vi "XY Graph Show-Hide Grid Event.vi"(8 "Error In":errorcluster, 11 "XYGraph in":T1) -> (0 "Error Out":errorcluster, 1 "Message":string)   [LabVIEW 2019, in "XY Graph Add-Ons.lvlib"]
uses:
  XY Graph Add-Ons.lvlib
  XY Graph Refnum.ctl
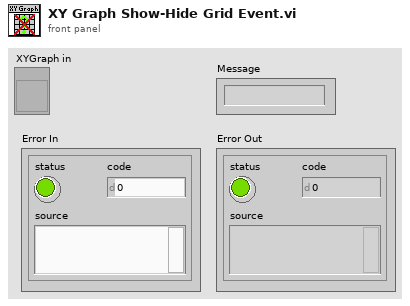
[diagram p1: front panel]
types:
  T1 = typedef "XY Graph Add-Ons.lvlib/XY Graph Refnum.ctl" = refnum<vi>
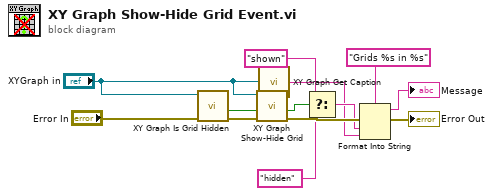
[diagram p0: block diagram]
diagram:
  n1 = call "XY Graph Is Grid Hidden.vi"("Error In"="Error In", "XY Graph Ref"="XYGraph in") -> ("Error Out (dup)"=w12:errorcluster, "Hidden Grid(s)"=w13:bool)  [unwired: 8 in]
  n2 = call "XY Graph Show-Hide Grid.vi"("Error In"=w12, "Hide (F) /Show (T)"=w13, "XY Graph Ref"="XYGraph in") -> ("Error Out"=w10:errorcluster, "Grid Shown?"=w6:bool)  [unwired: 7 in]
  n3 = call "XY Graph Get Caption.vi"("XYGraph"="XYGraph in") -> ("Graph Caption"=w1:string)  [unwired: 8 in]
  n4 = Select(t="shown" ("format string"), s=w6, f="hidden" ("format string")) -> (s? t:f=w3:string)
  n5 = Format Into String(format string="Grids %s in %s", error in=w10, w3, w1) -> (resulting string=→"Message":string, error out=→"Error Out":errorcluster)  [unwired: 1 in]
